vi "Read Sequencer State Machine.vi"(8 "error in (no error)":errorcluster, 11 "Simple Sequencer in":refnum<class "Simple Sequencer.lvclass">) -> (0 "error out":errorcluster, 2 "Sequencer State Machine.lvclass":refnum<class "Sequencer State Machine.lvclass">, 3 "Simple Sequencer out":refnum<class "Simple Sequencer.lvclass">)   [LabVIEW 2018, in "Simple Sequencer.lvclass"]
uses:
  Simple Sequencer.lvclass
  NHMFL_Core/Libraries/Instruments/Sequence/Sequencer State Machine/Sequencer State Machine.lvclass
  Simple Sequencer.lvclass/Simple Sequencer.ctl
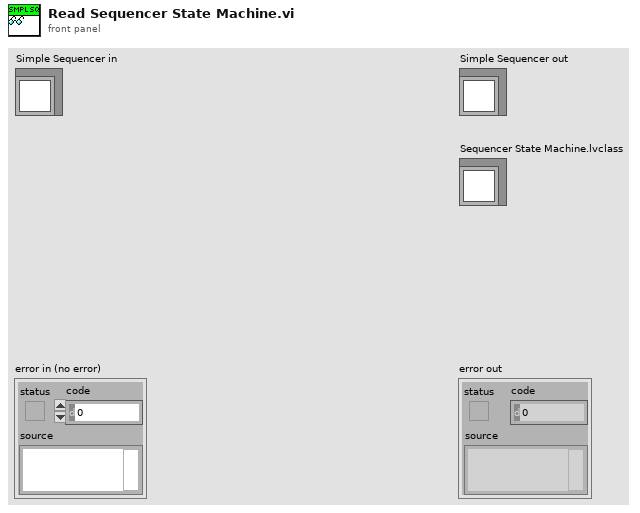
[diagram p1: front panel]
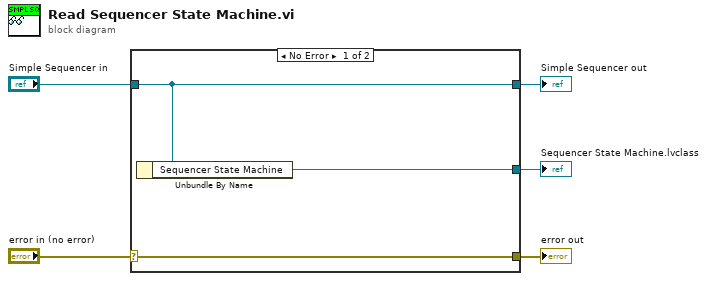
[diagram p0: block diagram]
diagram:
  n1 = case shown="No Error" "error in (no error)" {
    selector: "error in (no error)" -> [w8 w9]
    tunnel: [w8 w9] -> w4
    tunnel: [w7 w10] -> w2
    tunnel: "Simple Sequencer in" -> [w7 w10]
    tunnel: [w6 _] -> w1
    frame No Error {
      n2 = Unbundle By Name(w7) -> ("Sequencer State Machine"=w6:refnum<class "Sequencer State Machine.lvclass">)
    }
    frame Error {
    }
  }
  "error out" <- w4
  "Simple Sequencer out" <- w2
  "Sequencer State Machine.lvclass" <- w1
